vi "Add PV (String Array).vi"(6 "initial timestamp":timestamp, 7 "PV name":string, 8 "error in (no error)":errorcluster, 10 "initial value":string[](array[string]), 11 "Server in":refnum<class "Server.lvclass">) -> (0 "error out":errorcluster, 2 "value out":string[](array[string]), 3 "Server out":refnum<class "Server.lvclass">, 4 "timestamp out":timestamp)   [LabVIEW 2020, in "PV Access.lvlib" / "PVA Server.lvlib" / "Server.lvclass"]
uses:
  Server.lvclass
  PV Data/NT Scalar/NT Scalar.lvclass
  Server.lvclass/Server.ctl
  C:/Users/eyw68381/source/repos/pvaccess-labview/labview/source/PV Data/NT Base/NT Base.lvclass
  C:/Users/eyw68381/source/repos/pvaccess-labview/labview/source/PV Data/NT Scalar/NT Scalar.lvclass
  Source/Source.lvclass
  PV Data/PV Data.lvlib
  PV Data/NT Scalar/Create (String Array).vi
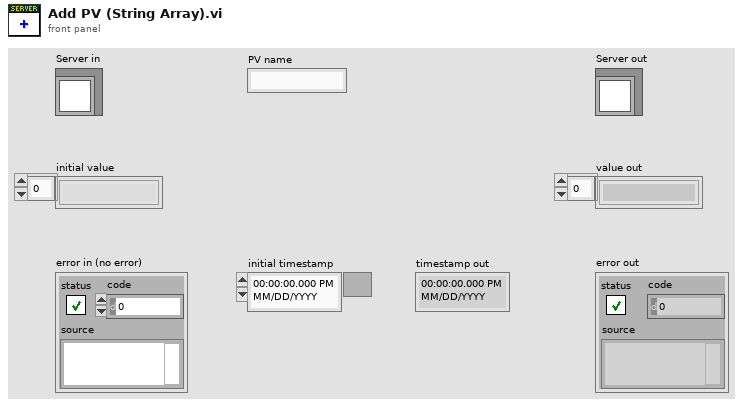
[diagram p1: front panel]
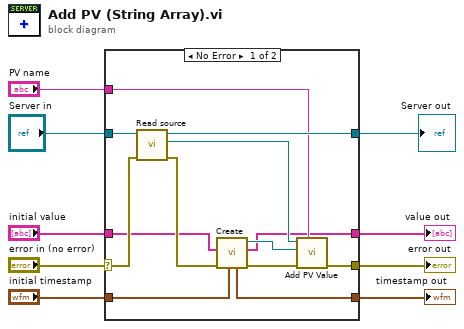
[diagram p0: block diagram]
diagram:
  n1 = case shown="No Error" "error in (no error)" {
    selector: "error in (no error)" -> [w18 w26]
    tunnel: [w17 w26] -> w8
    tunnel: [w21 w25] -> w6
    tunnel: "Server in" -> [w22 w25]
    tunnel: "PV name" -> [w19 _]
    tunnel: "initial value" -> [w13 w24]
    tunnel: [w12 w24] -> w3
    tunnel: "initial timestamp" -> [w11 w23]
    tunnel: [w10 w23] -> w1
    frame No Error {
      n2 = call "Read source.vi"("error in (no error)"=w18, "Server in"=w22) -> ("error out"=w16:errorcluster, "Source"=w20:refnum<class "Source.lvclass">, "Server out"=w21:refnum<class "Server.lvclass">)  [unwired: 7 in]
      n3 = call-poly "Create.vi"("timestamp in"=w11, "error in (no error)"=w16, "value in"=w13) -> ("error out"=w15:errorcluster, "value out"=w12:string[], "NT Scalar out"=w14:refnum<class "NT Scalar.lvclass">, "timestamp out"=w10:timestamp)  [unwired: 5 in]
      n4 = call "Add PV Value.vi"("PV name"=w19, "error in"=w15, "NT Base in"=w14, "Source in"=w20) -> ("error out"=w17:errorcluster)  [unwired: 5 in, 2 out]
    }
    frame Error {
    }
  }
  "error out" <- w8
  "Server out" <- w6
  "value out" <- w3
  "timestamp out" <- w1
